vi "Set Plot Color.vi"(8 "error in (no error)":errorcluster, 10 "Value":string, 11 "GraphChart in":refnum<vi>) -> (0 "error out":errorcluster)   [LabVIEW 2019, in "LSS.lvlib"]
doc: "Apply the desired color properties to either a Waveform Graph or Chart. Though LabVIEW uses two different property nodes to do this set, with LSS the same properties can be applied to both and this VI will determine which property node to use.\n\n<b>Inputs:</b>\n<b>GraphChart in</b> - Reference to the graph that will be set.\n<b>Value</b> - Value of the plot reference number and color.\n<b>Error In</b> - Standard Error in terminal.\n\n<b>Outputs:</b>\n<b>Error out</b> - Standard Error out terminal."
uses:
  LSS.lvlib
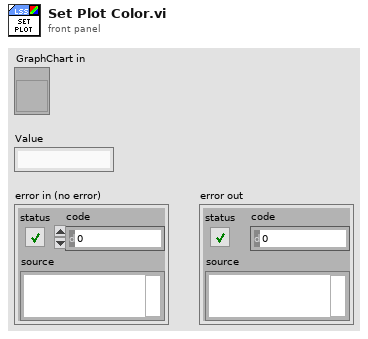
[diagram p1: front panel]
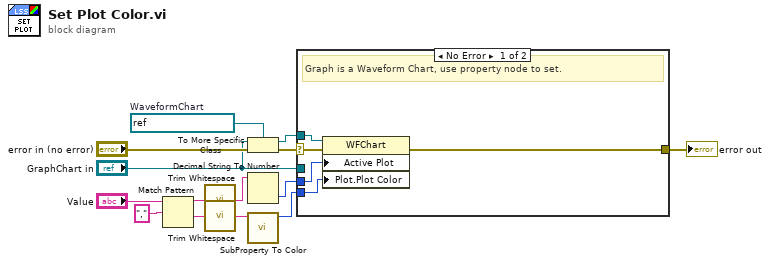
[diagram p0: block diagram]
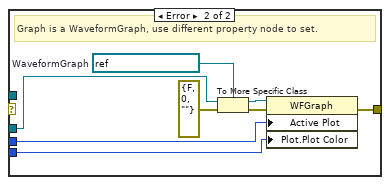
[diagram p2: hidden frame]
diagram:
  w7 = refnum<vi> refnum  # WaveformChart
  n1 = Match Pattern(string="Value", regular expression=",") -> (before substring=w11:string, after substring=w8:string)  [unwired: 1 in, 2 out]
  n2 = call <vilib>:"Trim Whitespace.vi"("string"=w11) -> ("trimmed string"=w13:string)  [unwired: 1 in]
  n3 = call <vilib>:"Trim Whitespace.vi"("string"=w8) -> ("trimmed string"=w10:string)  [unwired: 1 in]
  n4 = To More Specific Class(target class=w7, reference="GraphChart in", error in="error in (no error)") -> (specific class reference=w6:refnum<vi>, error out=w5:errorcluster)
  n5 = Decimal String To Number(string=w13) -> (number=w2:i32)  [unwired: 2 in, 1 out]
  n6 = call "SubProperty To Color.vi"("Value"=w10) -> ("Color"=w4:u32)  [unwired: 10 in]
  n7 = case shown="No Error" w5 {
    selector: w5 -> [w18 _]
    tunnel: w6 -> [w19 _]
    tunnel: w2 -> [w17 w24]
    tunnel: w4 -> [w16 w23]
    tunnel: [w15 w21] -> w3
    tunnel: "GraphChart in" -> [_ w20]
    frame No Error {
      # "Graph is a Waveform Chart, use property node to set."
      n8 = property class="WFChart"(reference=w19, error in=w18, "Active Plot"=w17, "Plot.Plot Color"=w16) -> (error out=w15:errorcluster)  [unwired: 1 out]
    }
    frame Error {
      w27 = refnum<vi> refnum  # WaveformGraph
      # "Graph is a WaveformGraph, use different property node to set."
      n9 = To More Specific Class(target class=w27, reference=w20, error in=errorcluster {"status"=FALSE, "code"=0, "source"=""}) -> (specific class reference=w26:refnum<vi>, error out=w25:errorcluster)
      n10 = property class="WFGraph"(reference=w26, error in=w25, "Active Plot"=w24, "Plot.Plot Color"=w23) -> (error out=w21:errorcluster)  [unwired: 1 out]
    }
  }
  "error out" <- w3
